vi "parse.series_reply.vi"(8 "error in":errorcluster, 11 "string in":string) -> (0 "error out":errorcluster, 3 "data":T1)   [LabVIEW 2024]
uses:
  TypeDefs/series.reply.ctl
  <vilib>/addons/_JKI.lib/Serialization/JSON/JKI JSON Serialization.lvlib
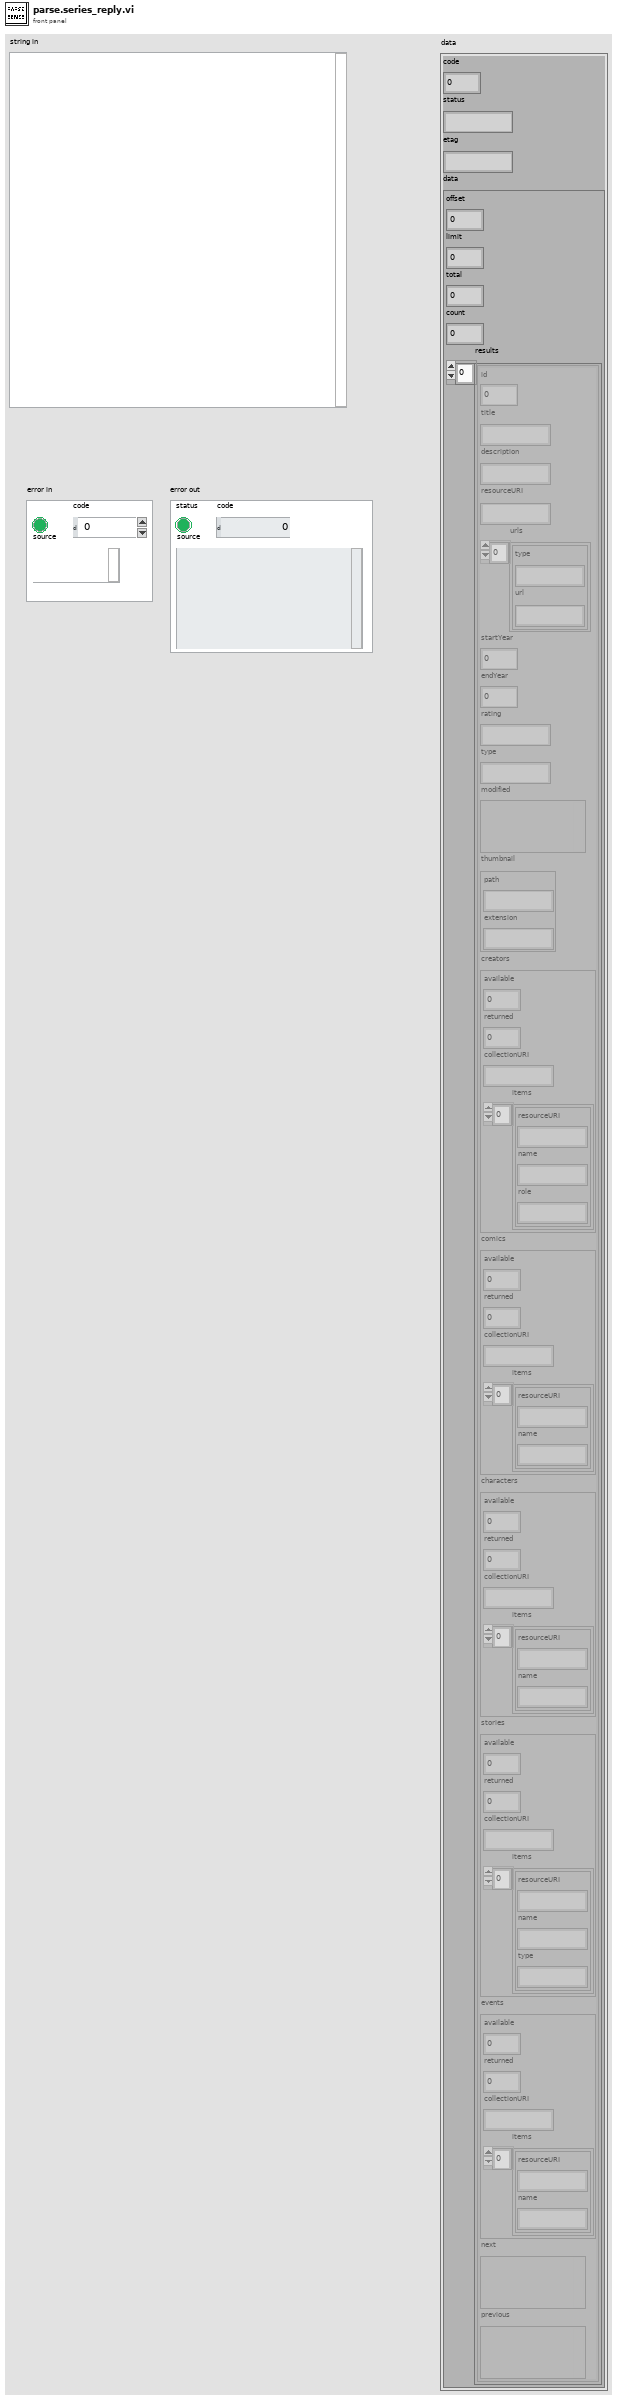
[diagram p1: front panel]
types:
  T1 = typedef "series.reply.ctl" = cluster{"code":i32, "status":string, "etag":string, "data":cluster{"offset":i32, "limit":i32, "total":i32, "count":i32, "results":cluster{"id":i32, "title":string, "description":string, "resourceURI":string, "urls":cluster{"type":string, "url":string}[], "startYear":i32, "endYear":i32, "rating":string, "type":string, "modified":variant, "thumbnail":cluster{"path":string, "extension":string}, "creators":cluster{"available":i32, "returned":i32, "collectionURI":string, "items":cluster{"resourceURI":string, "name":string, "role":string}[]}, "comics":cluster{"available":i32, "returned":i32, "collectionURI":string, "items":cluster{"resourceURI":string, "name":string}[]}, "characters":cluster{"available":i32, "returned":i32, "collectionURI":string, "items":cluster{"resourceURI":string, "name":string}[]}, "stories":cluster{"available":i32, "returned":i32, "collectionURI":string, "items":cluster{"resourceURI":string, "name":string, "type":string}[]}, "events":cluster{"available":i32, "returned":i32, "collectionURI":string, "items":cluster{"resourceURI":string, "name":string}[]}, "next":variant, "previous":variant}[]}}
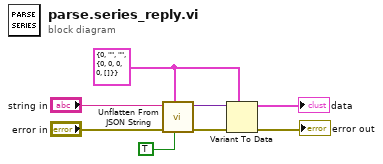
[diagram p0: block diagram]
diagram:
  w1 = T1 {"code"=0, "status"="", "etag"="", "data"={"offset"=0, "limit"=0, "total"=0, "count"=0, "results"=[]}} ("reply")
  n1 = call <vilib>:"Unflatten From JSON String.vi"("Nulls as Defaults (F)"=TRUE, "Type and Defaults"=w1, "error in"="error in", "JSON String"="string in") -> ("error out"=w5:errorcluster, "Variant"=w6:variant)  [unwired: 6 in]
  n2 = Variant To Data(error in=w5, type=w1, Variant=w6) -> (data=→"data":T1, error out=→"error out":errorcluster)
